vi "Read Unicode Text from File - Display as ASCII.vi"() -> ()   [LabVIEW 2009]
panel:
  out "File Contents (Hex)":string
  out "File Contents (Unicode Display)":string
  out "File Contents (ASCII Display)":string
  out "String":string caption="Greeting"
  # "ASCII String Indicator"
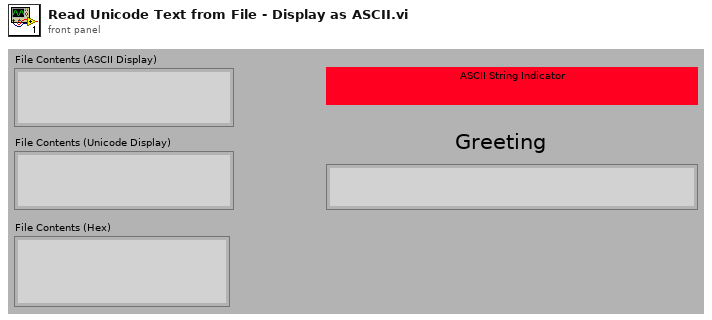
[diagram p1: front panel]
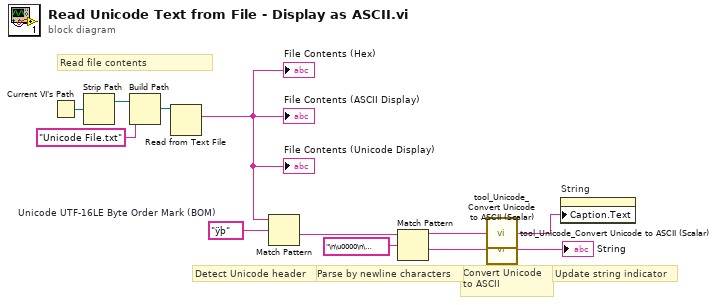
[diagram p0: block diagram]
diagram:
  w8 = "ÿþ"  # Unicode UTF-16LE Byte Order Mark (BOM)
  # "Update string indicator"
  # "Read file contents"
  # "Convert Unicode\nto ASCII"
  # "Parse by newline characters"
  # "Detect Unicode header"
  n1 = Current VI's Path() -> (path=w12:path)
  n2 = Strip Path(path=w12) -> (stripped path=w11:path)  [unwired: 1 out]
  n3 = Build Path(base path=w11, name or relative path="Unicode File.txt") -> (appended path=w9:path)
  n4 = Read from Text File(file (use dialog)=w9) -> (text=w5:string)  [unwired: 3 in, 3 out]
  "File Contents (ASCII Display)" <- w5
  "File Contents (Unicode Display)" <- w5
  "File Contents (Hex)" <- w5
  n5 = Match Pattern(string=w5, regular expression=w8) -> (after substring=w7:string)  [unwired: 1 in, 3 out]
  n6 = Match Pattern(string=w7, regular expression="\n\u0000\n\u0000") -> (before substring=w3:string, after substring=w4:string)  [unwired: 1 in, 2 out]
  n7 = call "tool_Unicode_Convert Unicode to ASCII (Scalar).vi"("Unicode"=w3) -> ("ASCII"=w2:string)  [unwired: 4 in]
  n8 = call "tool_Unicode_Convert Unicode to ASCII (Scalar).vi"("Unicode"=w4) -> ("ASCII"=→"String":string)  [unwired: 4 in]
  n9 = property on="String" class="Str"("Caption.Text"=w2) -> ()  [unwired: 2 in, 2 out]
